vi "Lesson 2-3 simple heart rate monitor.vi"() -> ()   [LabVIEW 2020]
uses:
  Lesson 1/HRM-AQN-input_clust.ctl
  <vilib>/measure/matone.llb/Extract Single Tone Information 1 Chan.vi
  <vilib>/measure/NI_MAPro.lvlib
panel:
  out "Heart Rate":dbl format="%.2p"
  out "detected frequency":dbl format="%.2p"
  in  "Additional Signal to remove [s]":i32
  out "Filtered data":waveform(dbl)(graph)
  in  "samples [s]":i32
  out "Raw collected data":waveform(dbl)(graph)
  out "error out":errorcluster
  in  "stop":bool
  out "Raw data":waveform(dbl)(graph)
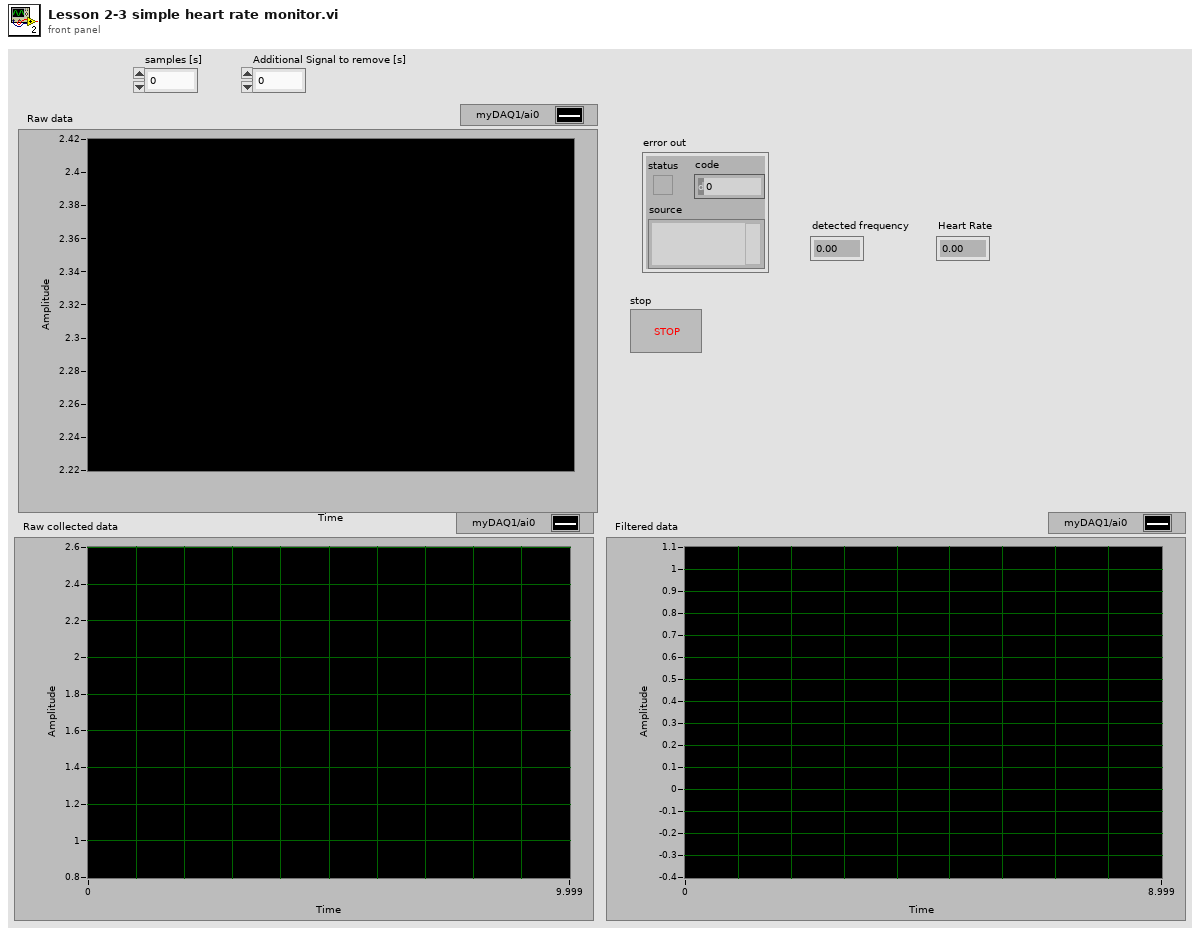
[diagram p1: front panel]
types:
  T1 = typedef "HRM-AQN-input_clust.ctl" = cluster{"physical channels":tag, "myDAQ task":refnum<k21>}
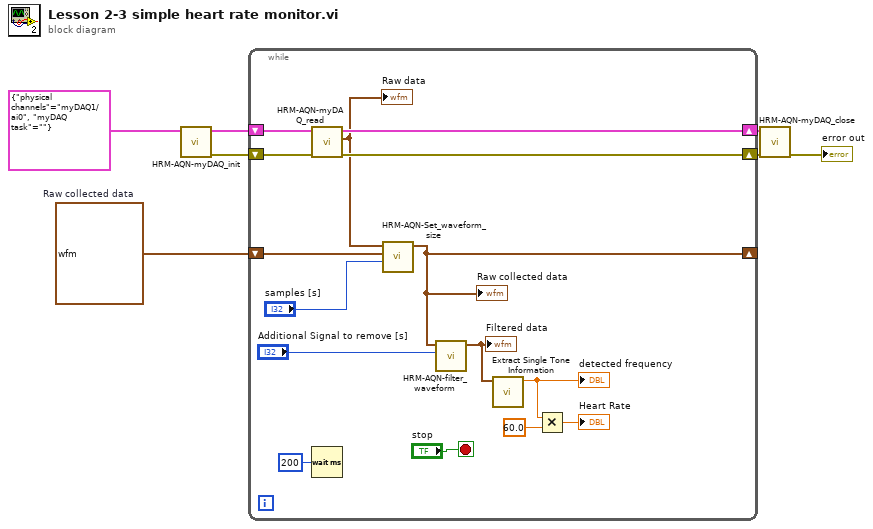
[diagram p0: block diagram]
diagram:
  w1 = waveform(dbl) {"t0"=timestamp(0 s since 1904-01-01), "dt"=1.0, "Y"=[]}  # Raw collected data
  n1 = call "HRM-AQN-myDAQ_init.vi"("AQN cluster in"=T1 {"physical channels"="myDAQ1/ai0", "myDAQ task"=""}) -> ("error out"=w7:errorcluster, "AQN cluster out"=w3:T1)  [unwired: 9 in]
  n2 = while {
    shift-right: [w17] -> w2
    shift-left: w3 -> [w18]
    shift-right: [w21] -> w6
    shift-left: w7 -> [w22]
    shift-right: [w13] -> _
    shift-left: w1 -> [w16]
    stop <- "stop" stop-if-true
    n3 = call "HRM-AQN-myDAQ_read.vi"("error in (no error)"=w22, "AQN cluster in"=w18) -> ("error out"=w21:errorcluster, "data"=w15:waveform(dbl), "AQN cluster out"=w17:T1)  [unwired: 7 in]
    "Raw data" <- w15
    n4 = Wait (ms)(milliseconds to wait=u32 200) -> ()  [unwired: 1 out]
    n5 = call "HRM-AQN-Set_waveform_size.vi"("samples [s]"="samples [s]", "Raw collected data"=w16, "data in"=w15) -> ("data out"=w13:waveform(dbl))  [unwired: 8 in]
    "Raw collected data" <- w13
    n6 = call "HRM-AQN-filter_waveform.vi"("Additional Signal to remove [s]"="Additional Signal to remove [s]", "data in"=w13) -> ("data out"=w11:waveform(dbl))  [unwired: 9 in]
    "Filtered data" <- w11
    n7 = call-poly <vilib>:"Extract Single Tone Information.vi"("time signal in"=w11) -> ("detected frequency"=w10:dbl)  [unwired: 5 in, 5 out]
    "detected frequency" <- w10
    n8 = Multiply(x=w10, y=60.0) -> (x*y=→"Heart Rate":dbl)
  }
  n9 = call "HRM-AQN-myDAQ_close.vi"("error in (no error)"=w6, "AQN cluster in"=w2) -> ("error out"=→"error out":errorcluster)  [unwired: 9 in]
